vi "Agilent PWM Send Command.vi"(7 "Read? (F)":bool, 8 "error in (no error)":errorcluster, 9 "Byte Count":u32, 10 "Command":string, 11 "VISA Resource Name":refnum<visa-resource-name>) -> (0 "error out":errorcluster, 2 "Data Read":string, 3 "dup VISA Resource Name":refnum<visa-resource-name>)   [LabVIEW 2011]
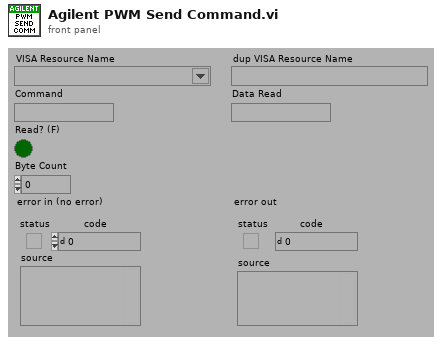
[diagram p1: front panel]
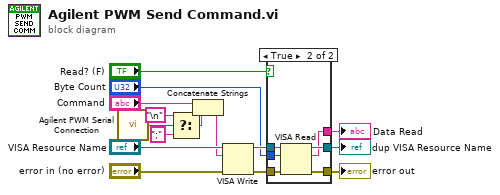
[diagram p0: block diagram]
diagram:
  n1 = call "Agilent PWM Serial Connection.vi"("VISA Resource Name"="VISA Resource Name") -> ("Serial?"=w13:bool)
  n2 = Select(t="\n", s=w13, f=";") -> (s? t:f=w10:string)
  n3 = Concatenate Strings("Command", w10) -> (w8:string)
  n4 = VISA Write(VISA resource name="VISA Resource Name", write buffer=w8, error in (no error)="error in (no error)") -> (VISA resource name out=w6:refnum<visa-resource-name>, error out=w7:errorcluster)  [unwired: 1 out]
  n5 = case shown="True" "Read? (F)" {
    tunnel: w7 -> [w16 w23]
    tunnel: w6 -> [w17 w22]
    tunnel: [w17 w21] -> w5
    tunnel: [w16 w20] -> w4
    tunnel: "Byte Count" -> [_ w19]
    tunnel: [_ w18] -> w1
    frame False {
    }
    frame True {
      n6 = VISA Read(VISA resource name=w22, byte count=w19, error in (no error)=w23) -> (VISA resource name out=w21:refnum<visa-resource-name>, read buffer=w18:string, error out=w20:errorcluster)  [unwired: 1 out]
    }
  }
  "error out" <- w4
  "dup VISA Resource Name" <- w5
  "Data Read" <- w1
